vi "HXQ-槽内铜碎-检测-MLin.vi"(6 "截图变量":T5, 8 "error in (no error)":errorcluster, 9 "检测控制参数和规范":T4={"从起始点向心偏移程度"=0.21999999999999997, "检槽宽度比例"=0.30000000000000004, "检槽高度比例"=0.2, "产品直径参考值"=900.0, "产品轴向角度_从底向上"=438.171, "SK槽宽上限"=40.0, "SK槽宽下限"=20.0}, 11 "ImageSRC":T2(plugin-control)) -> (0 "error out":errorcluster, 2 "铜碎检测OK":bool, 3 "Image Out":T2)   [LabVIEW 2018]
uses:
  <vilib>/vision/Measure.llb/Straight Edge Options.ctl
  <vilib>/vision/Measure.llb/Straight Edge Process.ctl
  <vilib>/vision/Measure.llb/Edge Options.ctl
  <vilib>/vision/Measure.llb/Edge Polarity.ctl
  <vilib>/vision/Image Controls.llb/IMAQ Image.ctl
  <vilib>/Analysis/coordinate.llb/Angle Units.ctl
  <vilib>/Analysis/coordinate.llb/Check for Included Angle (scalar).vi
  <vilib>/Analysis/coordinate.llb/Wrap Angle (scalar).vi
  <vilib>/Analysis/coordinate.llb/Absolute Angle Difference (scalar).vi
  <vilib>/Analysis/coordinate.llb/Set Angle Unit.vi
  <vilib>/vision/NI_Vision_Development_Module.lvlib
  <vilib>/Analysis/NI_AAL_Angle.lvlib
panel:
  in  "Selection Values (Particle Filter 1)":T1(array[cluster])=[{"Measurement Parameter"=35, "Range Lower Value"=0.0, "Range Upper Value"=200.0, "Range"=FALSE, "Measurement Type"=FALSE}] {"Measurement Parameter" items=["Center of Mass X", "Center of Mass Y", "First Pixel X", "First Pixel Y", "Bounding Rect Left", "Bounding Rect Top", "Bounding Rect Right", "Bounding Rect Bottom", "Max Feret Diameter Start X", "Max Feret Diameter Start Y", "Max Feret Diameter End X", "Max Feret Diameter End Y", "Max Horiz. Segment Length Left", "Max Horiz. Segment Length Right", "Max Horiz. Segment Length Row", "-", "Bounding Rect Width", "Bounding Rect Height", "Bounding Rect Diagonal", "Perimeter", "Convex Hull Perimeter", "Holes' Perimeter", "Max Feret Diameter", "Equivalent Ellipse Major Axis", "Equivalent Ellipse Minor Axis", "Equivalent Ellipse Minor Axis (Feret)", "Equivalent Rect Long Side", "Equivalent Rect Short Side", "Equivalent Rect Diagonal", "Equivalent Rect Short Side (Feret)", "Average Horiz. Segment Length", "Average Vert. Segment Length", "Hydraulic Radius", "Waddel Disk Diameter", "-", "Area", "Holes' Area", "Particle & Holes' Area", "Convex Hull Area", "Image Area", "-", "Number of Holes", "Number of Horiz. Segments", "Number of Vert. Segments", "-", "Orientation", "Max Feret Diameter Orientation", "-", "% Area/Image Area", "% Area/(Particle & Holes' Area)", "Ratio of Equivalent Ellipse Axes", "Ratio of Equivalent Rect Sides", "-", "Elongation Factor", "Compactness Factor", "Heywood Circularity Factor", "Type Factor", "-", "Sum X", "Sum Y", "Sum XX", "Sum XY", "Sum YY", "Sum XXX", "Sum XXY", "Sum XYY", "Sum YYY", "-", "Moment of Inertia XX", "Moment of Inertia XY", "Moment of Inertia YY", "Moment of Inertia XXX", "Moment of Inertia XXY", "Moment of Inertia XYY", "Moment of Inertia YYY", "Norm. Moment of Inertia XX", "Norm. Moment of Inertia XY", "Norm. Moment of Inertia YY", "Norm. Moment of Inertia XXX", "Norm. Moment of Inertia XXY", "Norm. Moment of Inertia XYY", "Norm. Moment of Inertia YYY", "Hu Moment 1", "Hu Moment 2", "Hu Moment 3", "Hu Moment 4", "Hu Moment 5", "Hu Moment 6", "Hu Moment 7"]}
  out "ImageReview 2":T2(plugin-control)
  out "白条检测OK":bool
  out "白条分析结果":dbl[][](array[numeric]) format="%.2f"
  in  "白条面积限度":T1(array[cluster])=[{"Measurement Parameter"=35, "Range Lower Value"=0.0, "Range Upper Value"=400.0, "Range"=FALSE, "Measurement Type"=FALSE}] {"Measurement Parameter" items=["Center of Mass X", "Center of Mass Y", "First Pixel X", "First Pixel Y", "Bounding Rect Left", "Bounding Rect Top", "Bounding Rect Right", "Bounding Rect Bottom", "Max Feret Diameter Start X", "Max Feret Diameter Start Y", "Max Feret Diameter End X", "Max Feret Diameter End Y", "Max Horiz. Segment Length Left", "Max Horiz. Segment Length Right", "Max Horiz. Segment Length Row", "-", "Bounding Rect Width", "Bounding Rect Height", "Bounding Rect Diagonal", "Perimeter", "Convex Hull Perimeter", "Holes' Perimeter", "Max Feret Diameter", "Equivalent Ellipse Major Axis", "Equivalent Ellipse Minor Axis", "Equivalent Ellipse Minor Axis (Feret)", "Equivalent Rect Long Side", "Equivalent Rect Short Side", "Equivalent Rect Diagonal", "Equivalent Rect Short Side (Feret)", "Average Horiz. Segment Length", "Average Vert. Segment Length", "Hydraulic Radius", "Waddel Disk Diameter", "-", "Area", "Holes' Area", "Particle & Holes' Area", "Convex Hull Area", "Image Area", "-", "Number of Holes", "Number of Horiz. Segments", "Number of Vert. Segments", "-", "Orientation", "Max Feret Diameter Orientation", "-", "% Area/Image Area", "% Area/(Particle & Holes' Area)", "Ratio of Equivalent Ellipse Axes", "Ratio of Equivalent Rect Sides", "-", "Elongation Factor", "Compactness Factor", "Heywood Circularity Factor", "Type Factor", "-", "Sum X", "Sum Y", "Sum XX", "Sum XY", "Sum YY", "Sum XXX", "Sum XXY", "Sum XYY", "Sum YYY", "-", "Moment of Inertia XX", "Moment of Inertia XY", "Moment of Inertia YY", "Moment of Inertia XXX", "Moment of Inertia XXY", "Moment of Inertia XYY", "Moment of Inertia YYY", "Norm. Moment of Inertia XX", "Norm. Moment of Inertia XY", "Norm. Moment of Inertia YY", "Norm. Moment of Inertia XXX", "Norm. Moment of Inertia XXY", "Norm. Moment of Inertia XYY", "Norm. Moment of Inertia YYY", "Hu Moment 1", "Hu Moment 2", "Hu Moment 3", "Hu Moment 4", "Hu Moment 5", "Hu Moment 6", "Hu Moment 7"]}
  out "铜碎检测特征值":sgl[](graph) caption="边沿检测LineProfile原始"
  out "ImageReview":T2(plugin-control)
  out "底边中心到拟合圆心连线":T3
  out "槽边夹角合规":bool
  out "正槽宽合规":bool
  out "SK槽宽":dbl format="%.2f"
  out "槽边线检测完成":bool
  out "修正后的起始点":cluster{dbl, dbl}
  in  "顶洞_RakeEdge Options 2":T6={"Edge Polarity"=0, "Kernel Size"=3, "Width"=9, "Minimum Edge Strength"=50.0, "Interpolation Type"=enum."Bilinear Fixed", "Data Processing Method"=enum."Average"} {"Edge Polarity" items=["All Edges", "Rising Edges", "Falling Edges"]; "Minimum Edge Strength" format="%.2f"; "Width" step=2; "Kernel Size" step=2}
  in  "高径比参数值":dbl=0.6
  out "边沿检测梯度":dbl[](graph)
  out "所得中线的端点属于正序":bool caption="范围内？"
  out "Angles (deg)":sgl[](array[numeric]) format="%.2f"
  in  "Edge Options横向槽边":T6={"Edge Polarity"=2, "Kernel Size"=5, "Width"=21, "Minimum Edge Strength"=40.0, "Interpolation Type"=enum."Bilinear Fixed", "Data Processing Method"=enum."Average"} {"Edge Polarity" items=["All Edges", "Rising Edges", "Falling Edges"]; "Minimum Edge Strength" format="%.2f"; "Width" step=2; "Kernel Size" step=2}
  in  "Line Options":T8={"Number of Lines"=1, "Type"=enum."First Edge Rake", "Min. Score"=100.0, "Max. Score"=1000.0, "Orientation"=0.0, "Angle Range"=10.0, "Angle Tolerance"=1.0, "Step Size"=5, "Min. SNR (db)"=0.0, "Min. Points (%)"=25.0, "Hough Iterations"=5} {"Min. Points (%)" min=0.0 max=100.0; "Min. SNR (db)" min=0.0; "Max. Score" min=0.0 max=1024.0; "Min. Score" min=0.0 max=1024.0 step=1.0}
  # "小洞，大洞：50,110"
  # "进行槽的横向边沿检测的时候\n最好对强度阈值进行动态自动配置，避免定值"
  # "槽的边沿强度需要认真设定，避免强度门槛太低引入干扰致找错位置。"
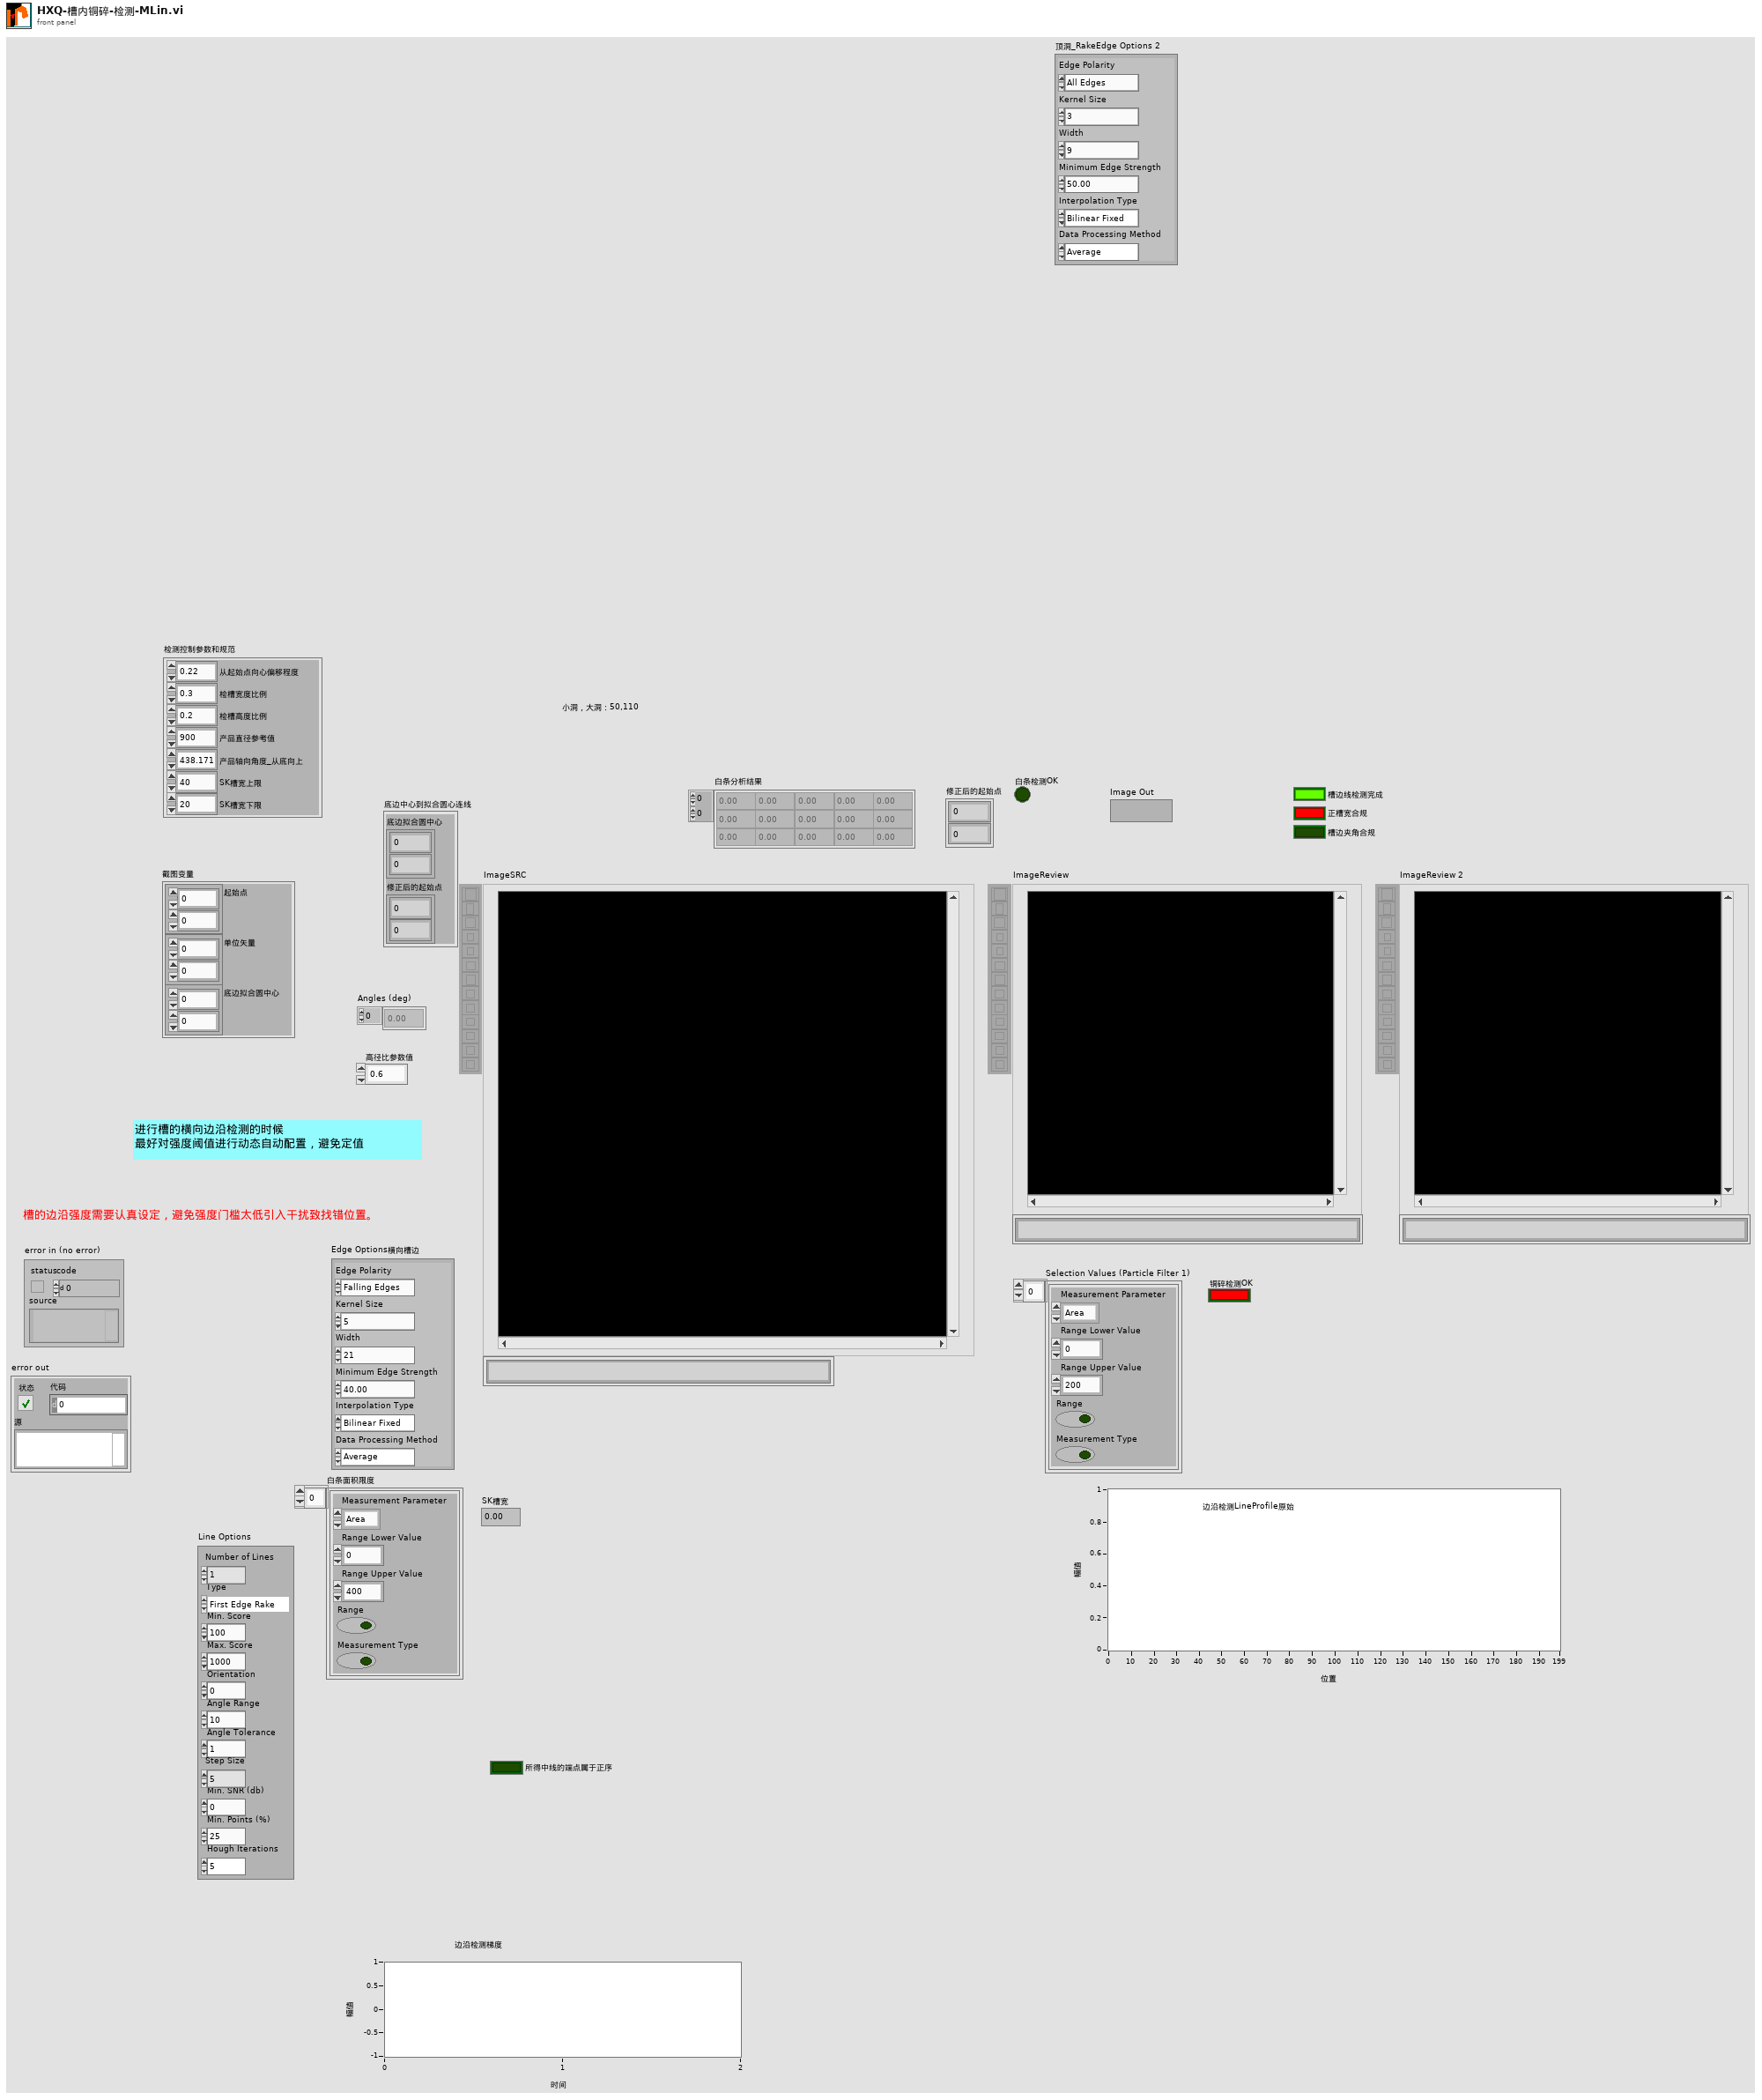
[diagram p1: front panel]
types:
  T1 = cluster{"Measurement Parameter":i32, "Range Lower Value":dbl, "Range Upper Value":dbl, "Range":bool, "Measurement Type":bool}[]
  T2 = typedef "IMAQ Image.ctl" = refnum<image>
  T3 = cluster{"底边拟合圆中心":cluster{dbl, dbl}, "修正后的起始点":cluster{dbl, dbl}}
  T4 = cluster{"从起始点向心偏移程度":dbl, "检槽宽度比例":dbl, "检槽高度比例":dbl, "产品直径参考值":dbl, "产品轴向角度_从底向上":dbl, "SK槽宽上限":dbl, "SK槽宽下限":dbl}
  T5 = cluster{"起始点":cluster{dbl, dbl}, "单位矢量":cluster{dbl, dbl}, "底边拟合圆中心":cluster{dbl, dbl}}
  T6 = typedef "Edge Options.ctl" = cluster{"Edge Polarity":T7, "Kernel Size":u32, "Width":u32, "Minimum Edge Strength":sgl, "Interpolation Type":enum32{"Zero Order", "Bilinear", "Quadratic", "Cubic", "Bilinear Fixed"}, "Data Processing Method":enum32{"Average", "Median"}}
  T7 = typedef "Edge Polarity.ctl" = u32
  T8 = typedef "Straight Edge Options.ctl" = cluster{"Number of Lines":i32, "Type":T9, "Min. Score":dbl, "Max. Score":dbl, "Orientation":dbl, "Angle Range":dbl, "Angle Tolerance":dbl, "Step Size":u32, "Min. SNR (db)":dbl, "Min. Points (%)":dbl, "Hough Iterations":i32}
  T9 = typedef "Straight Edge Process.ctl" = enum32{"First Edge Rake", "Best Edge Rake", "Hough Edge Rake", "First Edge Projection", "Best Edge Projection"}
  T10 = typedef "Image Type" = u32
  T11 = cluster{"起始点":cluster{dbl, dbl}, "单位矢量":cluster{dbl, dbl}, "产品直径参考值":dbl}
  T12 = typedef "IMAQ Rectangle" = cluster{"Left":i32, "Top":i32, "Right":i32, "Bottom":i32, "Rotation":dbl}
  T13 = typedef "ROI Descriptor" = cluster{"Global Rectangle":i32[], "Contours":cluster{"ID":enum32{"External", "Internal"}, "Type":u32, "Coordinates":i32[]}[]}
  T14 = cluster{"Point1 (Pixels)":cluster{"X":sgl, "Y":sgl}, "Point2 (Pixels)":cluster{"X":sgl, "Y":sgl}, "Point1 (Real-World)":cluster{"X":sgl, "Y":sgl}, "Point2 (Real-World)":cluster{"X":sgl, "Y":sgl}, "Angle (Pixel)":dbl, "Angle (Real-World)":dbl, "Score":dbl, "Straightness":dbl, "Average SNR (db)":dbl, "Calibration Valid":bool}[]
  T15 = cluster{"Point1 (Pixels)":cluster{"X":sgl, "Y":sgl}, "Point2 (Pixels)":cluster{"X":sgl, "Y":sgl}, "Point1 (Real-World)":cluster{"X":sgl, "Y":sgl}, "Point2 (Real-World)":cluster{"X":sgl, "Y":sgl}, "Angle (Pixel)":dbl, "Angle (Real-World)":dbl, "Score":dbl, "Straightness":dbl, "Average SNR (db)":dbl, "Calibration Valid":bool}
  T16 = cluster{"Point2 (Pixels)":cluster{"X":sgl, "Y":sgl}, "Point1 (Pixels)":cluster{"X":sgl, "Y":sgl}}
  T17 = typedef "IMAQ Line" = cluster{"Start X":i32, "Start Y":i32, "End X":i32, "End Y":i32}
  T18 = typedef "NI_AAL_Angle.lvlib/Angle Units.ctl" = i32
  T19 = cluster{"Point1 (Pixels)":cluster{"X":sgl, "Y":sgl}, "Point2 (Pixels)":cluster{"X":sgl, "Y":sgl}}
  T20 = cluster{"Point 1":cluster{"X":sgl, "Y":sgl}, "Point 2":cluster{"X":sgl, "Y":sgl}}
  T21 = cluster{"修正后的起始点":cluster{dbl, dbl}, "底边拟合圆中心":cluster{dbl, dbl}}
  T22 = typedef "IMAQ Point" = cluster{"X":sgl, "Y":sgl}
  T23 = cluster{"Interpolation Type":enum32{"Zero Order", "Bilinear", "Quadratic", "Cubic", "Bilinear Fixed"}, "Destination Width":u32, "Destination Height":u32, "Fill Value":sgl}
  T24 = typedef "IMAQ Circle" = cluster{"Center X":i32, "Center Y":i32, "Inner Radius":i32, "Outer Radius":i32, "Start Angle":dbl, "End Angle":dbl}
  T25 = enum16{"Get First Edge", "Get First + Last Edge", "Get All Edges", "Get Best Edge"}
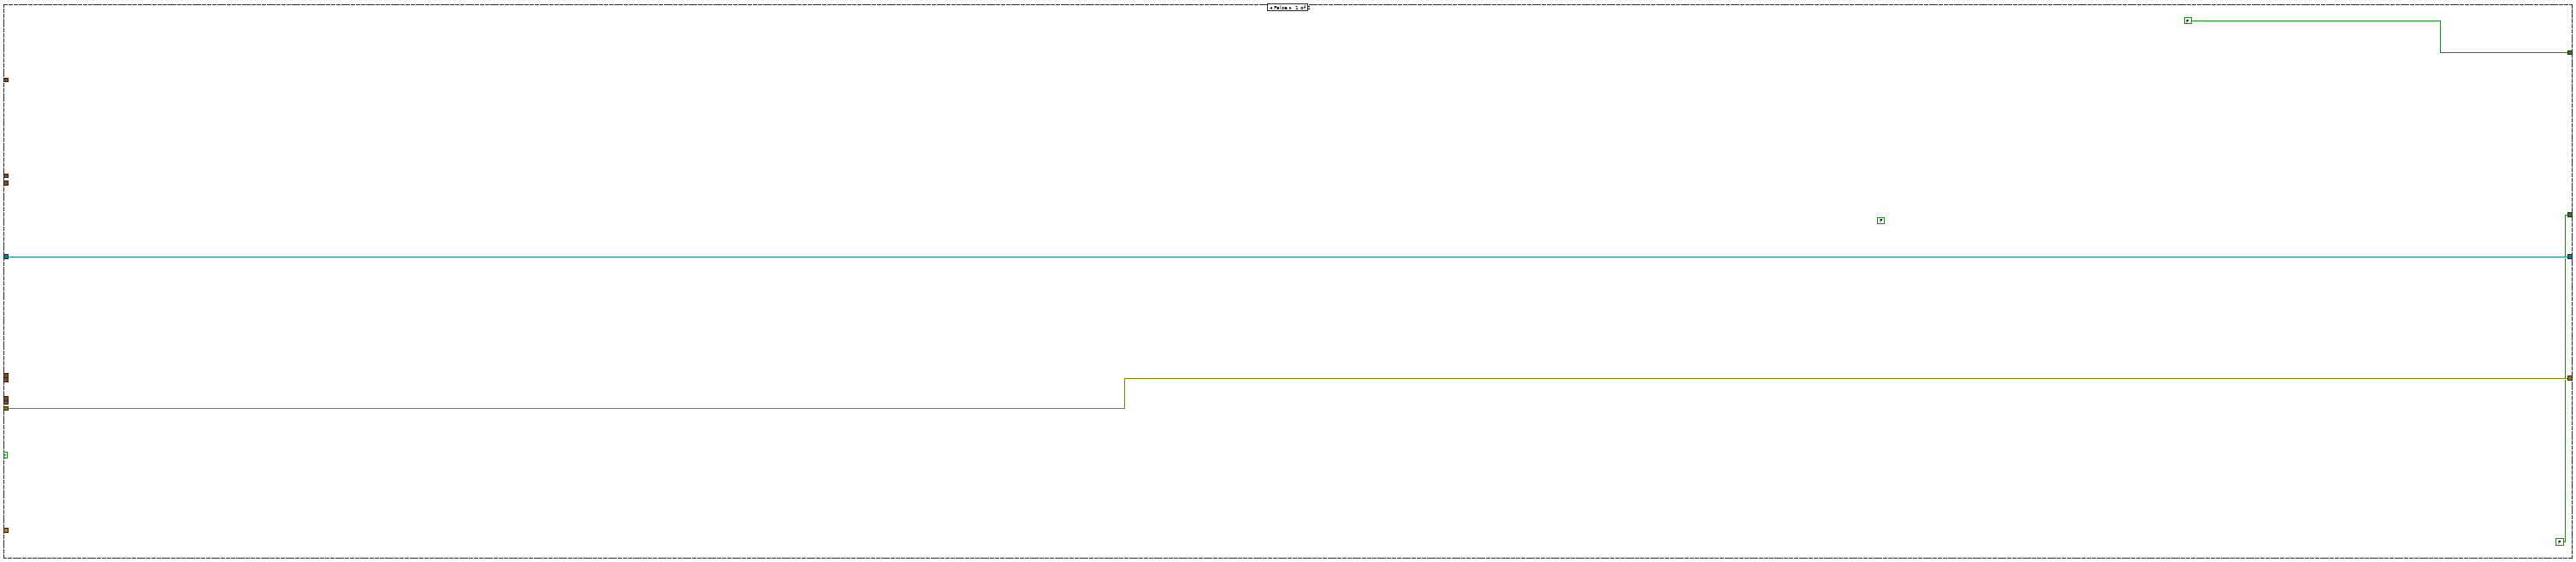
[diagram p8: hidden frame]
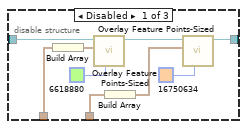
[diagram p14: hidden frame]
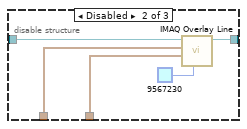
[diagram p15: hidden frame]
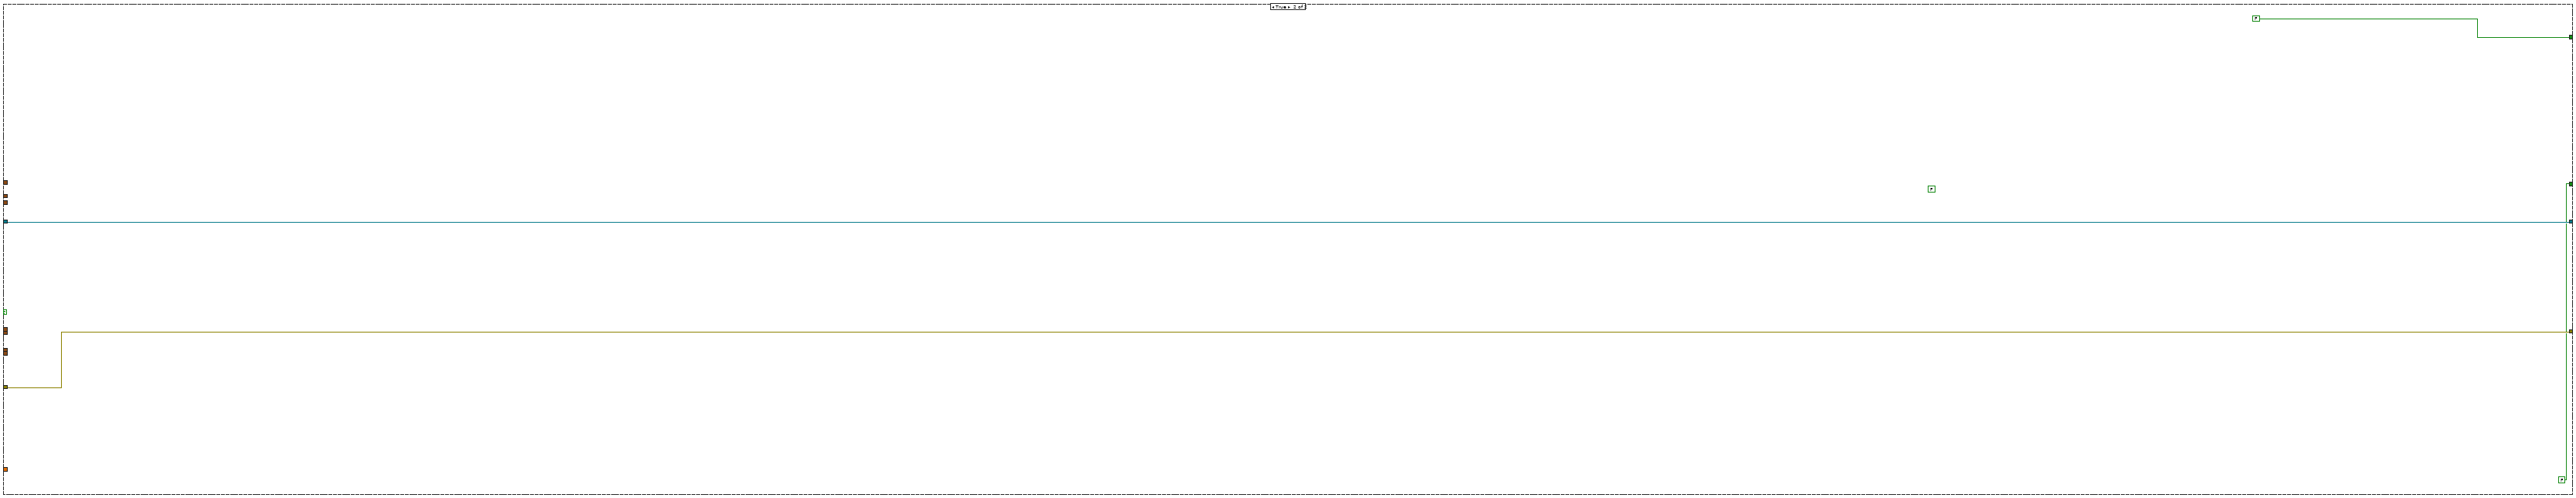
[diagram p17: hidden frame]
diagram:
  w12 = T10 4 items=["Grayscale (U8)", "Grayscale (I16)", "Grayscale (SGL)", "Complex (CSG)", "RGB (U32)", "HSL (U32)", "RGB (U64)", "Grayscale (U16)"] ("Image Type")
  w31 = u32 9567230  # 槽边线
  w55 = 0 ("索引")
  w60 = u32 3 items=["Left to Right", "Right to Left", "Top to Bottom", "Bottom to Top"] ("Search Direction")
  w61 = u32 2 items=["Left to Right", "Right to Left", "Top to Bottom", "Bottom to Top"] ("Search Direction")
  # "计算槽边线"
  # "计算其中一条线端点到另一条线的距离\n评估线间距的合规程度"
  # "起始点坐标+纵向偏移+横向偏移（起点/终点）"
  # "构造左右边界检测ROI，得到左右边界，对起始点作出修正"
  # "获取槽位的边沿强度，\n用以指导随后的边线搜索时边沿强度阈值"
  # "注意：如果外部裁切时遇到边界，则裁切的XY尺寸会发生异常，\n不能代表产品的半径，导致定位异常。"
  # "从大图中截取时，适当留出边际，以免检测底沿时遇到图像边界。"
  # "矩形ROI的大小，最好改为与底圆直径挂钩，以免后期调节（已挂钩）"
  n1 = Unbundle By Name("截图变量") -> ("底边拟合圆中心"=w18:cluster{dbl, dbl}, "起始点"=w22:cluster{dbl, dbl}, "单位矢量"=w17:cluster{dbl, dbl})
  n2 = call "IMAQ Clear Overlay"("error in (no error)"="error in (no error)", "Image"="ImageSRC") -> ("error out"=w69:errorcluster, "Image Out"=w71:T2)  [unwired: 8 in]
  n3 = Unbundle By Name("检测控制参数和规范") -> ("产品直径参考值"=w16:dbl, "从起始点向心偏移程度"=w26:dbl, "检槽宽度比例"=w25:dbl, "检槽高度比例"=w24:dbl, "产品轴向角度_从底向上"=w14:dbl)
  n4 = disable-structure shown="禁用" {
    frame Disabled {
      w88 = cluster{"X":sgl, "Y":sgl} {"X"=10.0, "Y"=10.0} ("y")
      n5 = Add(x=w88, y=cluster{"X":sgl, "Y":sgl} {"X"=1.0, "Y"=0.0}) -> (x+y=w92:cluster{"X":sgl, "Y":sgl})
      n6 = Build Array(w92, cluster{"X":sgl, "Y":sgl} {"X"=15.0, "Y"=5.0} ("y")) -> (w91:cluster{"X":sgl, "Y":sgl}[])
      n7 = call "IMAQ Get Angles"("Vertex"=w88, "Points"=w91, "Use Vertex (No)"=TRUE) -> ("Angles (deg)"=→"Angles (deg)":sgl[])  [unwired: 2 in, 2 out]
    }
    frame Enabled {
    }
  }
  n8 = Multiply(x=w16, y=w26) -> (x*y=w65:dbl)
  n9 = Multiply(x=w16, y=w25) -> (x*y=w64:dbl)
  n10 = Multiply(x=w16, y=w24) -> (x*y=w63:dbl)
  n11 = Multiply(x=w17, y=w65) -> (x*y=w67:cluster{dbl, dbl})
  n12 = Bundle("起始点"=w22, "单位矢量"=w17, "产品直径参考值"=w16) -> (w70:T11)  [unwired: 1 in]
  n13 = call "MLin-Skew-铜左右侧边界检测.vi"("error in (no error)"=w69, "位置参数"=w70, "ImgSrc"=w71) -> ("修正后的起始点"=w15:cluster{dbl, dbl}, "ImageOut"=w13:T2, "检测中部槽边横线"=w43:cluster{dbl, dbl, dbl, dbl})  [unwired: 3 in, 3 out]
  "修正后的起始点" <- w15
  n14 = Add(x=w15, y=w67) -> (x+y=w66:cluster{dbl, dbl})
  n15 = call "MLin-构造矩形区域1.vi"("转角"=w14, "高"=w63, "宽"=w64, "中心点"=w66) -> ("斜矩形"=w62:T12)  [unwired: 7 in]
  n16 = call "IMAQ Convert Line to ROI"("Line"=w43) -> ("ROI Descriptor"=w42:T13)  [unwired: 8 in, 1 out]
  n17 = call "IMAQ Convert Rectangle to ROI (Polygon)"("Rectangle"=w62) -> ("ROI Descriptor"=w40:T13)  [unwired: 7 in, 2 out]
  n18 = call "IMAQ Overlay ROI"("Colors (Green)"=u32[] [3381759], "ROI Descriptor"=w42, "Image"=w13) -> ("Image Out"=w41:T2)  [unwired: 7 in, 1 out]
  n19 = call "IMAQ Edge Tool 3"("Image"=w41, "Edge Options"="Edge Options横向槽边", "Optimized Mode"=FALSE, "ROI Descriptor"=w42) -> ("Image (duplicate)"=w72:T2, "Gradient Values"=w80:dbl[], "error out"=w45:errorcluster)  [unwired: 7 in, 2 out]
  n20 = Array Max & Min(array=w80) -> (max value=w79:dbl)  [unwired: 3 out]
  n21 = Multiply(x=w79, y=0.5) -> (x*y=w75:dbl)
  n22 = Bundle By Name(cluster="Edge Options横向槽边", "Minimum Edge Strength"=w75) -> (w76:T6)
  n23 = call "IMAQ Overlay ROI"("Colors (Green)"=u32[] [16860], "ROI Descriptor"=w40, "Image"=w72) -> ("Image Out"=w44:T2)  [unwired: 7 in, 1 out]
  n24 = call "IMAQ Find Straight Edges 3"("Image"=w44, "Edge Options"=w76, "ROI Descriptor"=w40, "Search Direction"=w61, "error in (no error)"=w45, "Line Options"="Line Options") -> ("Image (duplicate)"=w48:T2, "Straight Edges"=w54:T14, "error out"=w58:errorcluster)  [unwired: 5 in, 2 out]
  n25 = call "IMAQ Find Straight Edges 3"("Image"=w48, "Edge Options"=w76, "ROI Descriptor"=w40, "Search Direction"=w60, "error in (no error)"=w58, "Line Options"="Line Options") -> ("Image (duplicate)"=w20:T2, "Straight Edges"=w53:T14, "error out"=w51:errorcluster)  [unwired: 5 in, 2 out]
  n26 = Empty Array?(array=w54) -> (empty?=w50:bool)
  n27 = Empty Array?(array=w53) -> (empty?=w49:bool)
  n28 = call "IMAQ Overlay Line"("Color"=u32 3381759, "End Point"=w15, "Start Point"=w18, "Image"=w20) -> ("Image Out"=w19:T2)  [unwired: 6 in, 1 out]
  n29 = Compound Arithmetic op=OR ("复合运算")(w50, w49) -> (w74:bool)
  "槽边线检测完成" <- w74
  n30 = Index Array(array=w54, index=w55) -> (element=w57:T15)
  n31 = Index Array(array=w53, index=w55) -> (element=w56:T15)
  n32 = Unbundle By Name(w57) -> ("Point1 (Pixels)"=w35:cluster{"X":sgl, "Y":sgl}, "Point2 (Pixels)"=w34:cluster{"X":sgl, "Y":sgl})
  n33 = Unbundle By Name(w56) -> ("Point1 (Pixels)"=w33:cluster{"X":sgl, "Y":sgl}, "Point2 (Pixels)"=w32:cluster{"X":sgl, "Y":sgl})
  n34 = Unbundle By Name("检测控制参数和规范") -> ("SK槽宽上限"=w30:dbl, "SK槽宽下限"=w29:dbl)
  n35 = Bundle("Point2 (Pixels)"=w34, "Point1 (Pixels)"=w35) -> (w52:T16)  [unwired: 1 in]
  n36 = call "IMAQ Perpendicular Line"("error in (no error)"=w51, "Point"=w32, "Line"=w52) -> ("error out"=w46:errorcluster, "Distance"=w28:dbl)  [unwired: 6 in, 1 out]
  "SK槽宽" <- w28
  n37 = In Range and Coerce(upper limit=w30, x=w28, lower limit=w29) -> (In Range?=→"正槽宽合规":bool)  [unwired: 1 out]
  n38 = call <vilib>:"Clear Errors.vi"("error in (no error)"=w46) -> ("error out"=w73:errorcluster)  [unwired: 5 in, 1 out]
  n39 = call "IMAQ Overlay Line"("Color"=w31, "End Point"=w34, "Start Point"=w35, "Image"=w19) -> ("error out"=w39:errorcluster, "Image Out"=w38:T2)  [unwired: 6 in]
  n40 = call "IMAQ Overlay Line"("Color"=w31, "error in (no error)"=w39, "End Point"=w32, "Start Point"=w33, "Image"=w38) -> ("error out"=w36:errorcluster, "Image Out"=w37:T2)  [unwired: 5 in]
  n41 = Merge Errors(w36, w73) -> (w82:errorcluster)
  n42 = case shown="假" w74 {
    tunnel: w37 -> [w108 w360]
    tunnel: [w120 w360] -> w6
    tunnel: w82 -> [w117 w359]
    tunnel: [w111 w359] -> w4
    tunnel: w14 -> [w110 _]
    tunnel: w18 -> [w101 _]
    tunnel: w15 -> [w100 _]
    tunnel: w35 -> [w99 _]
    tunnel: w34 -> [w98 _]
    tunnel: w33 -> [w97 _]
    tunnel: w32 -> [w96 _]
    tunnel: [w95 FALSE] -> _
    tunnel: "检测控制参数和规范" -> [w94 _]
    tunnel: [w93 FALSE] -> w1
    frame False {
      w105 = u32 16860 ("Color")
      w102 = sgl 5.0  # 夹角允许值
      # "合规性检查：夹角小于特定值"
      n43 = call "IMAQ Overlay Line"("Color"=w105, "End Point"=w97, "Start Point"=w96, "Image"=w108) -> ("error out"=w106:errorcluster, "Image Out"=w107:T2)  [unwired: 6 in]
      n44 = call "IMAQ Overlay Line"("Color"=w105, "error in (no error)"=w106, "End Point"=w99, "Start Point"=w98, "Image"=w107) -> ("Image Out"=w109:T2)  [unwired: 5 in, 1 out]
      n45 = Build Array "确认边沿夹角正常"(w99, w98, w97, w96) -> (w121:cluster{"X":sgl, "Y":sgl}[])
      n46 = call "IMAQ Get Angles"("error in (no error)"=w117, "Points"=w121) -> ("error out"=w112:errorcluster, "Angles (deg)"=w119:sgl[])  [unwired: 3 in, 1 out]
      n47 = Index Array(array=w119, index=0 ("索引")) -> (element=w116:sgl)
      n48 = Subtract(x=sgl 360.0, y=w102) -> (x-y=w103:sgl)
      n49 = Less?(x=w116, y=w102) -> (x < y?=w115:bool)
      n50 = Greater?(x=w116, y=w103) -> (0:w114:bool)
      n51 = Or(x=w115, y=w114) -> (x .or. y?=w113:bool)
      "槽边夹角合规" <- w113
      n52 = case shown="真" w113 {
        tunnel: w99 -> [_ w275]
        tunnel: w98 -> [_ w274]
        tunnel: w97 -> [_ w273]
        tunnel: w96 -> [_ w272]
        tunnel: w109 -> [w125 w144]
        tunnel: [w125 w138] -> w120
        tunnel: w112 -> [w124 w268]
        tunnel: [w124 w192] -> w111
        tunnel: w110 -> [_ w261]
        tunnel: w101 -> [_ w150]
        tunnel: w100 -> [_ w151]
        tunnel: [FALSE FALSE] -> w95
        tunnel: w94 -> [_ w157]
        tunnel: [FALSE w126] -> w93
        frame False {
          (unwired) FALSE
        }
        frame True {
          w129 = T10 4 items=["Grayscale (U8)", "Grayscale (I16)", "Grayscale (SGL)", "Complex (CSG)", "RGB (U32)", "HSL (U32)", "RGB (U64)", "Grayscale (U16)"] ("Image Type")
          w148 = sgl -0.5  # 第二点向胶木方向延伸本长的比例
          w149 = sgl 0.5  # 第一点向铜底方向延伸比例
          w163 = "HXQCNTS_ROIs" ("字符串")
          w184 = "HXQCNTS_MASK" ("字符串")
          w215 = 0.01  # 扩展的槽区矩形半宽比例
          w216 = 0.25  # 槽区矩形半长比例
          w147 = sgl -0.1  # 向底部偏移比例
          w146 = sgl 0.5  # 中点因子
          w227 = 0.015  # 槽区矩形半宽比例
          w226 = 0.25  # 槽区矩形半长比例
          w209 = T12 {"Left"=0, "Top"=0, "Right"=0, "Bottom"=0, "Rotation"=0.0} ("Rectangle")
          w234 = cluster{"X":sgl, "Y":sgl} {"X"=1.0, "Y"=0.0}  # 构造X轴向
          w247 = T18 2 items=["弧度输入，弧度输出", "弧度输入，角度输出", "角度输入，角度输出", "角度输入，弧度输出"] ("angle units")
          w260 = 5.0 ("y")
          # "槽中间宽区有效，严格"
          # "槽中间窄区有效，宽松"
          # "计算槽中分线"
          # "这么繁琐的计算过程的原因是避免像素坐标的取整误差\n这个误差此处可能引入较大偏差"
          # "也可以通过测算，选择距离底部中点较近的点作为角度测量第三点"
          # "中分线端点远近次序不定，此处判断是否需要调序"
          n53 = Bundle("Point1 (Pixels)"=w275, "Point2 (Pixels)"=w274) -> (w271:T19)  [unwired: 1 in]
          n54 = Bundle("Point1 (Pixels)"=w273, "Point2 (Pixels)"=w272) -> (w270:T19)  [unwired: 1 in]
          n55 = call "IMAQ Bisecting Line"("error in (no error)"=w268, "Line 2"=w270, "Line 1"=w271) -> ("error out"=w132:errorcluster, "Bisecting Line"=w269:T20)  [unwired: 7 in]
          n56 = Bundle("修正后的起始点"=w151, "底边拟合圆中心"=w150) -> (→"底边中心到拟合圆心连线":T21)  [unwired: 1 in]
          n57 = Unbundle(w269) -> ("Point 1"=w254:cluster{"X":sgl, "Y":sgl}, "Point 2"=w253:cluster{"X":sgl, "Y":sgl})
          n58 = disable-structure shown="启用" {
            disable-tunnel: w144 -> [w340 w347 w348]
            disable-tunnel: w254 -> [w336 w345 _]
            disable-tunnel: w253 -> [w335 w344 _]
            disable-tunnel: [w334 w346 w348] -> w174
            frame Disabled {
              n59 = Build Array(w336) -> (w341:cluster{"X":sgl, "Y":sgl}[])
              n60 = call "Overlay Feature Points-Sized.vi"("Color"=u32 6618880, "Feature Points"=w341, "Image"=w340) -> ("Image Out"=w338:T2)  [unwired: 7 in, 1 out]
              n61 = Build Array(w335) -> (w337:cluster{"X":sgl, "Y":sgl}[])
              n62 = call "Overlay Feature Points-Sized.vi"("Color"=u32 16750634, "Feature Points"=w337, "Image"=w338) -> ("Image Out"=w334:T2)  [unwired: 7 in, 1 out]
            }
            frame Disabled {
              n63 = call "IMAQ Overlay Line"("Color"=u32 9567230, "End Point"=w344, "Start Point"=w345, "Image"=w347) -> ("Image Out"=w346:T2)  [unwired: 6 in, 1 out]
            }
            frame Enabled {
            }
          }
          n64 = Random Number (0-1)() -> (number: 0 to 1=w203:dbl)
          n65 = Add(x=w254, y=cluster{"X":sgl, "Y":sgl} {"X"=1.0, "Y"=0.0}) -> (x+y=w265:cluster{"X":sgl, "Y":sgl})
          n66 = Build Array(w265, w253) -> (w264:cluster{"X":sgl, "Y":sgl}[])
          n67 = Multiply(x=w203, y=100000000.0) -> (x*y=w201:dbl)
          n68 = To Unsigned Long Integer(number=w201) -> (unsigned 32bit integer=w196:u32)
          n69 = call "IMAQ Get Angles"("Vertex"=w254, "Points"=w264, "Use Vertex (No)"=TRUE) -> ("Angles (deg)"=w263:sgl[])  [unwired: 2 in, 2 out]
          n70 = Increment(x=w196) -> (x+1=w193:u32)
          n71 = Index Array(array=w263, index=0 ("索引")) -> (element=w256:sgl)
          n72 = Number To Hexadecimal String(2:w196) -> (0:w200:string)  [unwired: 1 in]
          n73 = Increment(x=w193) -> (x+1=w185:u32)
          n74 = Add(x=w261, y=w260) -> (x+y=w258:dbl)
          n75 = Number To Hexadecimal String(2:w193) -> (0:w197:string)  [unwired: 1 in]
          n76 = Subtract(x=w261, y=w260) -> (x-y=w259:dbl)
          n77 = Subtract(x=360.0, y=w256) -> (x-y=w255:dbl)
          n78 = Increment(x=w185) -> (x+1=w186:u32)
          n79 = Increment(x=w185) -> (x+1=w175:u32)
          n80 = Number To Hexadecimal String(2:w185) -> (0:w195:string)  [unwired: 1 in]
          n81 = call-poly <vilib>:"Check for Included Angle.vi"("angle units"=w247, "end angle"=w258, "start angle"=w259, "angle in"=w255) -> ("in range?"=w252:bool)  [unwired: 5 in, 2 out]
          "所得中线的端点属于正序" <- w252
          n82 = Unbundle(w254) -> ("X"=w251:sgl, "Y"=w250:sgl)
          n83 = Unbundle(w253) -> ("X"=w249:sgl, "Y"=w248:sgl)
          n84 = Increment(x=w175) -> (x+1=w162:u32)
          n85 = Number To Hexadecimal String(2:w186) -> (0:w187:string)  [unwired: 1 in]
          n86 = Number To Hexadecimal String(2:w175) -> (0:w189:string)  [unwired: 1 in]
          n87 = Increment(x=w162) -> (x+1=w161:u32)
          n88 = Number To Hexadecimal String(2:w162) -> (0:w177:string)  [unwired: 1 in]
          n89 = Concatenate Strings(w184, w200) -> (w199:string)
          n90 = Concatenate Strings(w184, w197) -> (w198:string)
          n91 = Concatenate Strings(w184, w195) -> (w194:string)
          n92 = Concatenate Strings(w184, w187) -> (w188:string)
          n93 = case "调整中线端点顺序" shown="真" w252 {
            tunnel: w251 -> [w352 w356]
            tunnel: [w350 w356] -> w246
            tunnel: [w349 w355] -> w245
            tunnel: w250 -> [w351 w355]
            tunnel: [w352 w354] -> w244
            tunnel: w249 -> [w350 w354]
            tunnel: [w351 w353] -> w243
            tunnel: w248 -> [w349 w353]
            frame False {
            }
            frame True {
            }
          }
          n94 = Unbundle By Name(w157) -> ("产品直径参考值"=w156:dbl)
          n95 = Number To Hexadecimal String(2:w161) -> (0:w164:string)  [unwired: 1 in]
          n96 = call "IMAQ Create"("Image Name"=w199, "Image Type"=w129) -> ("New Image"=w137:T2)  [unwired: 3 in, 1 out]
          n97 = call "IMAQ Create"("Image Name"=w198) -> ("New Image"=w141:T2)  [unwired: 4 in, 1 out]
          n98 = call "IMAQ Create"("Image Name"=w194) -> ("New Image"=w140:T2)  [unwired: 4 in, 1 out]
          n99 = call "IMAQ Create"("Image Name"=w188) -> ("New Image"=w183:T2)  [unwired: 4 in, 1 out]
          n100 = Bundle("X"=w246, "Y"=w245) -> (w225:cluster{"X":sgl, "Y":sgl})  [unwired: 1 in]
          n101 = Bundle("X"=w244, "Y"=w243) -> (w170:cluster{"X":sgl, "Y":sgl})  [unwired: 1 in]
          n102 = Concatenate Strings(w163, w189) -> (w190:string)
          n103 = Concatenate Strings(w163, w177) -> (w176:string)
          n104 = Concatenate Strings(w163, w164) -> (w165:string)
          n105 = call "IMAQ Create"("Image Name"=w190) -> ("New Image"=w182:T2)  [unwired: 4 in, 1 out]
          n106 = call "IMAQ Create"("Image Name"=w176) -> ("New Image"=w155:T2)  [unwired: 4 in, 1 out]
          n107 = call "IMAQ Create"("Image Name"=w165) -> ("New Image"=w160:T2)  [unwired: 4 in, 1 out]
          n108 = Add(x=w225, y=w170) -> (x+y=w224:cluster{"X":sgl, "Y":sgl})
          n109 = Subtract(x=w225, y=w170) -> (x-y=w173:cluster{"X":sgl, "Y":sgl})
          n110 = Add(x=w234, y=w225) -> (x+y=w235:cluster{"X":sgl, "Y":sgl})
          n111 = Multiply "取中点"(x=w224, y=w146) -> (x*y=w223:cluster{"X":sgl, "Y":sgl})
          n112 = Multiply ("x")(x=w173, y=w147) -> (x*y=w222:cluster{"X":sgl, "Y":sgl})
          n113 = Multiply(x=w173, y=w149) -> (x*y=w242:cluster{"X":sgl, "Y":sgl})
          n114 = Multiply(x=w173, y=w148) -> (x*y=w171:cluster{"X":sgl, "Y":sgl})
          n115 = Build Array(w235, w170) -> (w236:cluster{"X":sgl, "Y":sgl}[])
          n116 = Add(x=w225, y=w242) -> (x+y=w241:cluster{"X":sgl, "Y":sgl})
          n117 = Add(x=w170, y=w171) -> (x+y=w169:cluster{"X":sgl, "Y":sgl})
          n118 = disable-structure shown="启用" {
            disable-tunnel: w241 -> [w316 _]
            disable-tunnel: w170 -> [w315 _]
            disable-tunnel: w174 -> [w313 w317]
            disable-tunnel: [w312 w317] -> w166
            frame Enabled {
              n119 = call "IMAQ Overlay Line"("Color"=u32 16711680, "End Point"=w316, "Start Point"=w315, "Image"=w313) -> ("Image Out"=w312:T2)  [unwired: 6 in, 1 out]
            }
            frame Disabled {
            }
          }
          n120 = Add(x=w223, y=w222) -> (x+y=w221:cluster{"X":sgl, "Y":sgl})
          n121 = call "IMAQ Get Angles"("Vertex"=w225, "Points"=w236, "Use Vertex (No)"=TRUE) -> ("Angles (deg)"=w237:sgl[])  [unwired: 2 in, 2 out]
          n122 = Multiply(x=w156, y=w216) -> (x*y=w214:dbl)
          n123 = Multiply(x=w156, y=w215) -> (x*y=w218:dbl)
          n124 = Multiply(x=w156, y=w226) -> (x*y=w228:dbl)
          n125 = Multiply(x=w156, y=w227) -> (x*y=w219:dbl)
          n126 = Unbundle "选框中心点"(w221) -> ("X"=w208:sgl, "Y"=w207:sgl)
          n127 = Unbundle(w241) -> ("X"=w179:sgl, "Y"=w178:sgl)
          n128 = Unbundle(w169) -> ("X"=w168:sgl, "Y"=w167:sgl)
          n129 = Index Array(array=w237, index=0 ("索引")) -> (element=w240:sgl)
          n130 = Add(x=w208, y=w214) -> (x+y=w212:dbl)
          n131 = Add(x=w208, y=w228) -> (x+y=w230:dbl)
          n132 = Subtract(x=w208, y=w214) -> (x-y=w210:dbl)
          n133 = Subtract(x=w208, y=w228) -> (x-y=w232:dbl)
          n134 = Bundle(cluster=T17 {"Start X"=0, "Start Y"=0, "End X"=0, "End Y"=0} ("Line"), "Start X"=w179, "Start Y"=w178, "End X"=w168, "End Y"=w167) -> (w180:T17)
          n135 = Subtract "槽中线角度"(x=360.0, y=w240) -> (x-y=w159:dbl)
          n136 = Subtract(x=w207, y=w218) -> (x-y=w211:dbl)
          n137 = Add(x=w207, y=w218) -> (x+y=w213:dbl)
          n138 = Subtract(x=w207, y=w219) -> (x-y=w231:dbl)
          n139 = Add(x=w207, y=w219) -> (x+y=w229:dbl)
          n140 = call "IMAQ Convert Line to ROI"("error in (no error)"=w132, "Line"=w180) -> ("error out"=w133:errorcluster, "ROI Descriptor"=w143:T13)  [unwired: 7 in]
          n141 = Bundle By Name "制作搜边选框"(cluster=w209, "Left"=w210, "Top"=w211, "Right"=w212, "Bottom"=w213, "Rotation"=w159) -> (w217:T12)
          n142 = Bundle By Name "制作搜边选框"(cluster=w209, "Left"=w232, "Top"=w231, "Right"=w230, "Bottom"=w229, "Rotation"=w159) -> (w139:T12)
          n143 = call "IMAQ Overlay ROI"("Colors (Green)"=u32[] [9567230], "error in (no error)"=w133, "ROI Descriptor"=w143, "Image"=w166) -> ("error out"=w153:errorcluster, "Image Out"=w154:T2)  [unwired: 6 in]
          n144 = call "IMAQ Convert Rectangle to ROI (Polygon)"("Rectangle"=w139) -> ("Rectangle Points"=w130:T22[], "ROI Descriptor"=w131:T13)  [unwired: 7 in, 1 out]
          n145 = call "IMAQ Convert Rectangle to ROI (Polygon)"("Rectangle"=w217) -> ("ROI Descriptor"=w158:T13)  [unwired: 7 in, 2 out]
          n146 = call "IMAQ Overlay ROI"("Colors (Green)"=u32[] [13168384], "error in (no error)"=w153, "ROI Descriptor"=w131, "Image"=w154) -> ("error out"=w204:errorcluster, "Image Out"=w205:T2)  [unwired: 6 in]
          n147 = call "IMAQ Overlay ROI"("Colors (Green)"=u32[] [14429696], "error in (no error)"=w204, "ROI Descriptor"=w158, "Image"=w205) -> ("error out"=w134:errorcluster, "Image Out"=w138:T2)  [unwired: 6 in]
          n148 = disable-structure shown="禁用" {
            frame Disabled {
              (unwired) T23 {"Interpolation Type"=enum."Bilinear Fixed", "Destination Width"=100, "Destination Height"=100, "Fill Value"=0.0} ("Options")
              (unwired) cluster{"x":sgl, "y":sgl}[] [{"x"=100.0, "y"=100.0}, {"x"=200.0, "y"=100.0}, {"x"=200.0, "y"=200.0}, {"x"=100.0, "y"=200.0}] ("Tetragon")
              n149 = Index Array(index #1=0 ("索引"), index #2=1 ("索引"), index #3=2 ("索引"), index #4=3 ("索引")) -> (element #1=w279, element #2=w278, element #3=w277, element #4=w276)  [unwired: 1 in]
              n150 = Build Array(w279, w278, w277, w276) -> ()  [unwired: 1 out]
            }
            frame Enabled {
            }
          }
          n151 = call-poly "IMAQ Extract Tetragon"("error in (no error)"=w134, "Tetragon"=w130, "Image Dst"=w137, "Image Src"=w138) -> ("error out"=w135:errorcluster, "Image Dst Out"=w136:T2)  [unwired: 6 in]
          n152 = call "铜碎分析"("Image In"=w136, "Selection Values (Particle Filter 1)"="Selection Values (Particle Filter 1)", "error in"=w135) -> ("Number of Particles (Particle Analysis 1)"=w127:i32, "error out"=w142:errorcluster)  [unwired: 21 in, 2 out]
          n153 = Equal To 0?(x=w127) -> (x = 0?=w126:bool)
          n154 = disable-structure shown="禁用" {
            frame Disabled {
              n155 = call "MLin-Skew-头缺分析1.vi"() -> ()  [unwired: 12 in]
            }
            frame Enabled {
            }
          }
          n156 = disable-structure shown="禁用" {
            disable-tunnel: w141 -> [w311 _]
            disable-tunnel: w138 -> [w307 _]
            frame Disabled {
              w303 = T10 4 items=["Grayscale (U8)", "Grayscale (I16)", "Grayscale (SGL)", "Complex (CSG)", "RGB (U32)", "HSL (U32)", "RGB (U64)", "Grayscale (U16)"] ("Image Type")
              n157 = call "白条分析"("Image In"=w307, "Image Dst"=w311, "Selection Values (Particle Filter 1)"="白条面积限度") -> ("Particle Measurements (Pixels) (Particle Analysis 1)"=w309:dbl[][])  [unwired: 22 in, 2 out]
              "白条分析结果" <- w309
              n158 = Empty Array?(array=w309) -> (empty?=→"白条检测OK":bool)
              n159 = Call Chain() -> (call chain=w298:string[])
              n160 = Index Array(array=w298) -> (element=w299:string)  [unwired: 1 in]
              n161 = Concatenate Strings("IMGReview" ("Backup Image Name"), " ", w299) -> (w302:string)
              n162 = call "IMAQ Create"("Image Name"=w302, "Image Type"=w303) -> ("New Image"=w297:T2)  [unwired: 2 in, 2 out]
              n163 = call "脏污分析"("Image In"=w307, "Image Dst"=w297) -> ("Image Out"=w306:T2)  [unwired: 24 in, 1 out]
              n164 = call "IMAQ Multiply"("Image Src A"=w306, "Constant"=255.0) -> ("Image Dst Out"=→"ImageReview 2":T2)  [unwired: 5 in, 1 out]
            }
            frame Enabled {
            }
          }
          n165 = disable-structure shown="禁用" {
            disable-tunnel: [w285 _] -> _
            frame Disabled {
              w286 = 10  # 铜碎检测限度
              n166 = Unbundle By Name() -> ("Pixels Line"=w289:sgl[])  [unwired: 1 in]
              "铜碎检测特征值" <- w289
              n167 = property on="铜碎检测特征值" class="WFChart (严格)"("History Data"=sgl[] [] ("历史数据")) -> ()  [unwired: 2 in, 2 out]
              n168 = for {
                tunnel: w289 -> [w296] mode=indexing
                shift-right: [w290] -> w287
                shift-left: 0 -> [w293]
                n169 = Not Equal To 0?(x=w296) -> (x != 0?=w295:bool)
                n170 = Select(t=1, s=w295, f=0) -> (s? t:f=w294:i32)
                n171 = Add(x=w294, y=w293) -> (x+y=w290:i32)
              }
              n172 = Less?(x=w287, y=w286) -> (x < y?=w285:bool)
            }
            frame Enabled {
            }
          }
          n173 = flat-sequence {
            tunnel: w142 -> [w318]
            tunnel: [w318] -> w191
            tunnel: w137 -> [w333]
            tunnel: w141 -> [w332]
            tunnel: w140 -> [w331]
            tunnel: [w320] -> w192
            tunnel: w191 -> [w322]
            tunnel: w183 -> [w326]
            tunnel: w182 -> [w325]
            tunnel: w155 -> [w323]
            tunnel: w160 -> [w319]
            frame #0 {
            }
            frame #1 {
              n174 = call "IMAQ Dispose"("Image"=w333, "error in (no error)"=w322) -> ("error out"=w330:errorcluster)  [unwired: 4 in]
              n175 = call "IMAQ Dispose"("Image"=w332, "error in (no error)"=w330) -> ("error out"=w329:errorcluster)  [unwired: 4 in]
              n176 = call "IMAQ Dispose"("Image"=w331, "error in (no error)"=w329) -> ("error out"=w327:errorcluster)  [unwired: 4 in]
              n177 = call "IMAQ Dispose"("Image"=w326, "error in (no error)"=w327) -> ("error out"=w328:errorcluster)  [unwired: 4 in]
              n178 = call "IMAQ Dispose"("Image"=w325, "error in (no error)"=w328) -> ("error out"=w324:errorcluster)  [unwired: 4 in]
              n179 = call "IMAQ Dispose"("Image"=w323, "error in (no error)"=w324) -> ("error out"=w321:errorcluster)  [unwired: 4 in]
              n180 = call "IMAQ Dispose"("Image"=w319, "error in (no error)"=w321) -> ("error out"=w320:errorcluster)  [unwired: 4 in]
            }
          }
        }
      }
    }
    frame True {
      (unwired) FALSE
    }
  }
  "铜碎检测OK" <- w1
  "Image Out" <- w6
  n181 = disable-structure shown="禁用" {
    frame Disabled {
    }
    frame Enabled {
    }
  }
  n182 = disable-structure shown="禁用" {
    disable-tunnel: _ -> [w379 _]
    disable-tunnel: [w378 _] -> _
    disable-tunnel: _ -> [w374 _]
    disable-tunnel: _ -> [w366 _]
    disable-tunnel: _ -> [w364 _]
    frame Disabled {
      w368 = 5.0 ("y")
      w382 = u16 0 items=["Outside To Inside", "Inside To Outside"] ("Scan Direction")
      n183 = Unbundle By Name(w379) -> ("Center (Pixels).X"=w376, "Center (Pixels).Y"=w375, "Radius (Pixels)"=w369)
      n184 = Unbundle By Name(w374) -> ("Start Angle"=w373, "End Angle"=w372)
      n185 = Subtract(x=w369, y=w368) -> (x-y=w370:dbl)
      n186 = Add(x=w369, y=w368) -> (x+y=w371:dbl)
      n187 = Bundle By Name(cluster=T24 {"Center X"=0, "Center Y"=0, "Inner Radius"=0, "Outer Radius"=0, "Start Angle"=0.0, "End Angle"=0.0} ("Annulus 2"), "Center X"=w376, "Center Y"=w375, "Start Angle"=w373, "End Angle"=w372, "Inner Radius"=w370, "Outer Radius"=w371) -> (w367:T24)
      n188 = call "IMAQ Convert Annulus to ROI"("Annulus"=w367) -> ("ROI Descriptor"=w363:T13)  [unwired: 8 in, 1 out]
      n189 = call "IMAQ Overlay ROI"("Colors (Green)"=u32[] [10813184], "error in (no error)"=w366, "ROI Descriptor"=w363, "Image"=w364) -> ("error out"=w365:errorcluster, "Image Out"=w361:T2)  [unwired: 6 in]
      n190 = call "IMAQ Spoke 4"("Image"=w361, "Edge Options"="顶洞_RakeEdge Options 2", "ROI Descriptor"=w363, "Scan Direction"=w382, "error in (no error)"=w365, "Process"=T25."Get First Edge") -> ("error out"=w378:errorcluster)  [unwired: 6 in, 3 out]
    }
    frame Enabled {
    }
  }
  n191 = Call Chain() -> (call chain=w7:string[])
  n192 = disable-structure shown="禁用" {
    frame Disabled {
      n193 = call "Vision Assistant2"() -> ()  [unwired: 26 in, 2 out]
    }
    frame Enabled {
    }
  }
  n194 = Index Array(array=w7) -> (element=w8:string)  [unwired: 1 in]
  n195 = disable-structure shown="禁用" {
    disable-tunnel: _ -> [w393 _]
    disable-tunnel: _ -> [w392 _]
    disable-tunnel: _ -> [w391 _]
    disable-tunnel: _ -> [w390 _]
    disable-tunnel: _ -> [w384 _]
    disable-tunnel: [w383 _] -> _
    frame Disabled {
      w385 = u32 16738816 ("Text Color (black)")
      n196 = call "IMAQ Overlay Text"("Text Color (black)"=w385, "String"="1", "Origin"=w393, "Image"=w384) -> ("Image Out"=w396:T2)  [unwired: 6 in, 1 out]
      n197 = call "IMAQ Overlay Text"("Text Color (black)"=w385, "String"="2", "Origin"=w392, "Image"=w396) -> ("Image Out"=w395:T2)  [unwired: 6 in, 1 out]
      n198 = call "IMAQ Overlay Text"("Text Color (black)"=w385, "String"="3", "Origin"=w391, "Image"=w395) -> ("Image Out"=w394:T2)  [unwired: 6 in, 1 out]
      n199 = call "IMAQ Overlay Text"("Text Color (black)"=w385, "String"="4", "Origin"=w390, "Image"=w394) -> ("Image Out"=w383:T2)  [unwired: 6 in, 1 out]
    }
    frame Enabled {
    }
  }
  n200 = Concatenate Strings("IMGReview" ("Backup Image Name"), " ", w8) -> (w11:string)
  n201 = call "IMAQ Create"("Image Name"=w11, "Image Type"=w12) -> ("New Image"=w5:T2)  [unwired: 2 in, 2 out]
  n202 = call "IMAQ Copy"("error in (no error)"=w4, "Image Dst"=w5, "Image Src"=w6) -> ("error out"=→"error out":errorcluster, "Image Dst Out"=→"ImageReview":T2)  [unwired: 3 in]
  n203 = disable-structure shown="禁用" {
    disable-tunnel: _ -> [w397 _]
    frame Disabled {
      n204 = call "Vision Assistant"("Image In"=w397) -> ()  [unwired: 25 in, 2 out]
    }
    frame Enabled {
    }
  }
